vi "Write.Buffer.vi"(8 "error in (no error)":errorcluster, 9 "Offset":i32, 10 "Values":dbl[](array[numeric]), 11 "Write in":refnum<class "Write.lvclass">) -> (0 "error out":errorcluster, 3 "Write out":refnum<class "Write.lvclass">)   [LabVIEW 2015, in "Data Access Engine.lvlib" / "Write.lvclass"]
uses:
  Write.lvclass
  Write.lvclass/Write.ctl
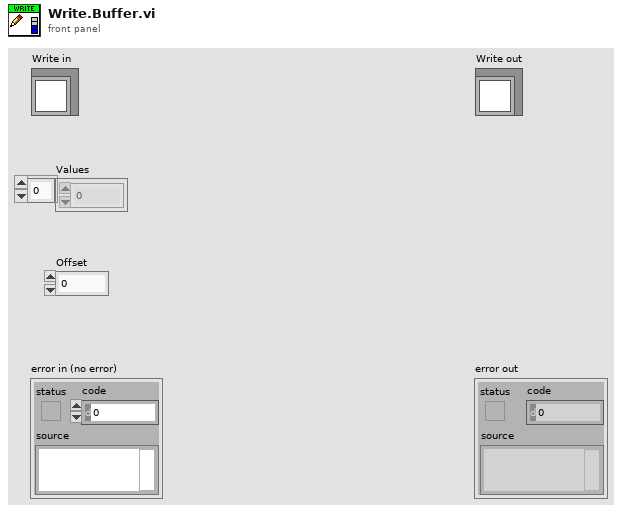
[diagram p1: front panel]
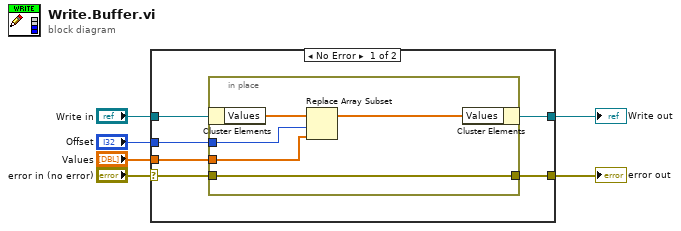
[diagram p0: block diagram]
diagram:
  n1 = case shown="No Error" "error in (no error)" {
    selector: "error in (no error)" -> [w10 w19]
    tunnel: [w9 w19] -> w5
    tunnel: [w11 w18] -> w3
    tunnel: "Write in" -> [w12 w18]
    tunnel: "Offset" -> [w8 _]
    tunnel: "Values" -> [w7 _]
    frame No Error {
      n2 = in-place {
        in-place-border: w7 -> [w17]
        in-place-border: w10 -> [w13]
        in-place-border: [w13] -> w9
        in-place-border: w8 -> [w14]
        n3 = in-place-cluster #1(w12) -> ("Values"=w16:dbl[])
        n4 = Replace Array Subset(array=w16, new element=w17, index=w14) -> (w15:dbl[])
        n5 = in-place-cluster #1("Values"=w15) -> (w11:refnum<class "Write.lvclass">)
      }
    }
    frame Error {
    }
  }
  "error out" <- w5
  "Write out" <- w3
